vi "Configure Triggered Voltage Mode.vi"(8 "error in (no error)":errorcluster {"code" format="%.0x"}, 9 "Voltage Mode (0: Fixed)":i32(ring) items=["Fixed", "Step", "List", "Waveform"], 10 "Channel Name (1)":string="1", 11 "VISA resource name":refnum<visa-resource-name>) -> (0 "error out":errorcluster {"code" format="%.0x"}, 3 "VISA resource name out":refnum<visa-resource-name>)   [LabVIEW 2016, in "Agilent N6700 Series.lvlib"]
doc: "Configures the power supply what happens to the output voltage when the transient system is initiated and triggered."
uses:
  <instrlib>/Agilent N6700 Series/Agilent N6700 Series.lvlib
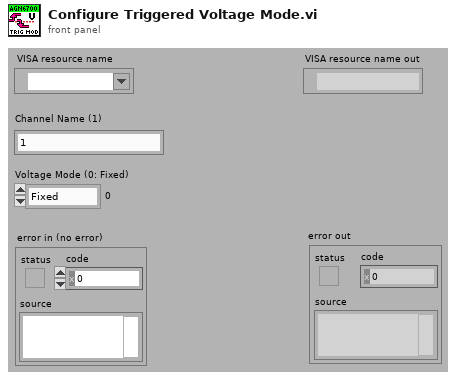
[diagram p1: front panel]
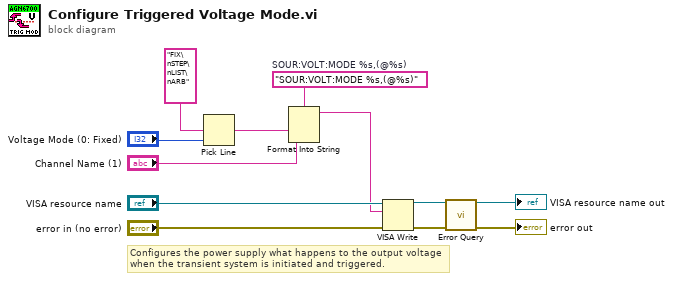
[diagram p0: block diagram]
diagram:
  w12 = "SOUR:VOLT:MODE %s,(@%s)"  # SOUR:VOLT:MODE %s,(@%s)
  # "Configures the power supply what happens to the output voltage \nwhen the transient system is initiated and triggered."
  n1 = Pick Line(multi-line string="FIX\nSTEP\nLIST\nARB", line index="Voltage Mode (0: Fixed)") -> (output string=w10:string)  [unwired: 1 in]
  n2 = Format Into String(format string=w12, w10, "Channel Name (1)") -> (resulting string=w6:string)  [unwired: 2 in, 1 out]
  n3 = VISA Write(VISA resource name="VISA resource name", write buffer=w6, error in (no error)="error in (no error)") -> (VISA resource name out=w2:refnum<visa-resource-name>, error out=w1:errorcluster)  [unwired: 1 out]
  n4 = call <instrlib>:"Error Query.vi"("VISA resource name"=w2, "error in (no error)"=w1) -> ("VISA resource name out"=→"VISA resource name out":refnum<visa-resource-name>, "error out"=→"error out":errorcluster)  [unwired: 10 in, 2 out]
